vi "PUB.vi"() -> ()   [LabVIEW 2018]
uses:
  Channel Pub/Channel Pub.lvclass
  C:/Users/Denis/Desktop/communication-manager/communication-manager/Communication Channel/Communication Channel.lvclass
  RxTx/RxTx.lvclass
  <vilib>/addons/zeromq/zmq_context.lvclass
  Communication Channel/Communication Channel.lvclass
panel:
  in  "Send":bool
  in  "Message":string
  out "error out":errorcluster
  in  "RxTx in":refnum<class "RxTx.lvclass">
  in  "Stop App":bool
  in  "Channel Pub.lvclass":refnum<class "Channel Pub.lvclass">
  # "PUBLISH example"
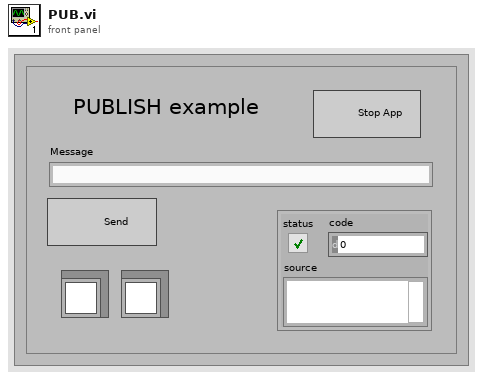
[diagram p1: front panel]
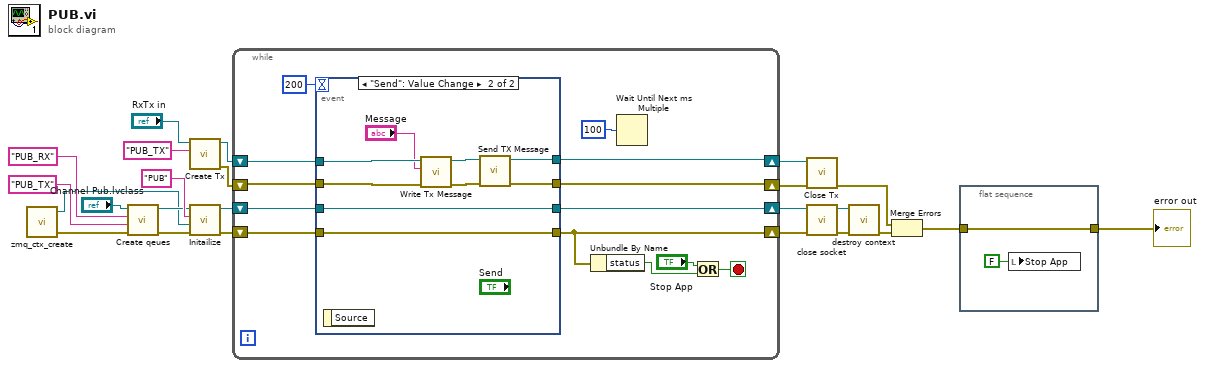
[diagram p0: block diagram]
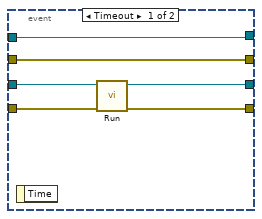
[diagram p2: hidden frame]
diagram:
  n1 = call <vilib>:"zmq_ctx_create.vi"() -> ("error out"=w24:errorcluster, "context out"=w5:refnum<class "zmq_context.lvclass">)  [unwired: 4 in]
  n2 = call "Create qeues.vi"("error in (no error)"=w24, "name qeue Tx"="PUB_TX" ("name qeue Rx"), "name qeue Rx"="PUB_RX", "Communication Channel in"="Channel Pub.lvclass") -> ("error out"=w17:errorcluster, "Communication Channel out"=w18:refnum<class "Channel Pub.lvclass">)  [unwired: 6 in]
  n3 = call "Create Tx.vi"("Writer Name"="PUB_TX", "RxTx in"="RxTx in") -> ("error out"=w12:errorcluster, "RxTx out"=w13:refnum<class "RxTx.lvclass">)  [unwired: 8 in]
  n4 = call-dynamic "Initailize.vi"("error in (no error)"=w17, "zeromq.lvlib:ZeroMQ Context"=w5, "Name"="PUB", "Channel Pub in"=w18) -> ("error out"=w22:errorcluster, "Channel Pub out"=w23:refnum<class "Channel Pub.lvclass">)  [unwired: 6 in]
  n5 = while {
    shift-right: [w35] -> w20
    shift-left: w23 -> [w37]
    shift-right: [w33] -> w19
    shift-left: w22 -> [w36]
    shift-right: [w28] -> w10
    shift-left: w13 -> [w29]
    shift-right: [w26] -> w9
    shift-left: w12 -> [w27]
    stop <- w30 stop-if-true
    n6 = event shown="[1] \"Send\": Value Change" {
      selector: _ -> [_ _]
      dyn-events: _ -> [_ _]
      timeout: 200 -> [_ _]
      tunnel: w37 -> [w43 w52]
      tunnel: w36 -> [w42 w51]
      tunnel: [w41 w52] -> w35
      tunnel: [w40 w51] -> w33
      tunnel: w29 -> [w39 w48]
      tunnel: [w39 w50] -> w28
      tunnel: w27 -> [w38 w45]
      tunnel: [w38 w49] -> w26
      event Timeout {
        n7 = event-data() -> ()  [unwired: 1 in, 1 out]
        n8 = call-dynamic "Run.vi"("error in (no error)"=w42, "Channel Pub in"=w43) -> ("error out"=w40:errorcluster, "Channel Pub out"=w41:refnum<class "Channel Pub.lvclass">)  [unwired: 8 in]
      }
      event "Send": Value Change {
        n9 = event-data() -> ()  [unwired: 1 in, 1 out]
        n10 = call "Write Tx Message.vi"("error in (no error)"=w45, "Tx Message"="Message", "RxTx in"=w48) -> ("error out"=w46:errorcluster, "RxTx out"=w47:refnum<class "RxTx.lvclass">)  [unwired: 7 in]
        n11 = call "Send TX Message.vi"("error in (no error)"=w46, "RxTx in"=w47) -> ("error out"=w49:errorcluster, "RxTx out"=w50:refnum<class "RxTx.lvclass">)  [unwired: 8 in]
      }
    }
    n12 = Unbundle By Name(w33) -> ("status"=w32:bool)
    n13 = Wait Until Next ms Multiple(millisecond multiple=u32 100) -> ()  [unwired: 1 out]
    n14 = Or(x="Stop App", y=w32) -> (x .or. y?=w30:bool)
  }
  n15 = call "Close Tx.vi"("error in (no error)"=w9, "RxTx in"=w10) -> ("error out"=w4:errorcluster)  [unwired: 8 in, 1 out]
  n16 = call "close socket.vi"("error in (no error)"=w19, "Communication Channel in"=w20) -> ("error out"=w7:errorcluster, "Communication Channel out"=w6:refnum<class "Channel Pub.lvclass">)  [unwired: 8 in]
  n17 = call "destroy context.vi"("error in (no error)"=w7, "Communication Channel in"=w6) -> ("error out"=w3:errorcluster)  [unwired: 8 in, 1 out]
  n18 = Merge Errors(w4, w3) -> (w2:errorcluster)
  n19 = flat-sequence {
    tunnel: w2 -> [w54]
    tunnel: [w54] -> w1
    frame #0 {
      n20 = local write "Stop App"(FALSE ("Stop App")) -> ()
    }
  }
  "error out" <- w1
